vi "Set_positions_speeds.vi"(0 "m1":dbl, 1 "m2":dbl, 2 "m3":dbl, 3 "m4":dbl, 4 "m5":dbl, 5 "m6":dbl, 7 "error in (no error)":errorcluster, 9 "Speed m1":dbl, 11 "Speed m2":dbl, 13 "Speed m3":dbl, 15 "Speed m4":dbl, 17 "Speed m5":dbl, 19 "Speed m6":dbl) -> (27 "error out":errorcluster)   [LabVIEW 2017]
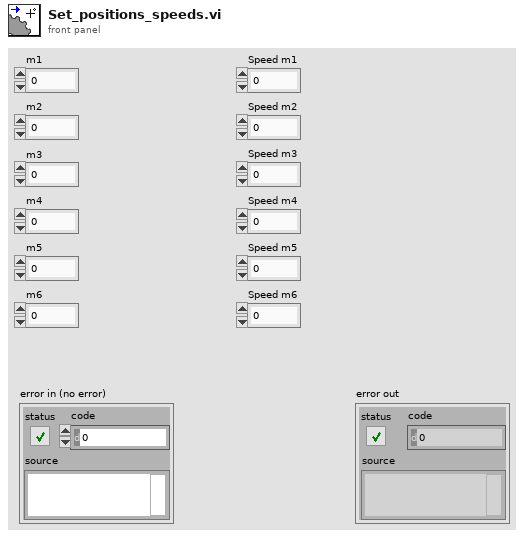
[diagram p1: front panel]
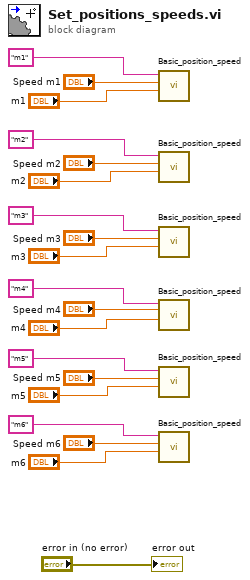
[diagram p0: block diagram]
diagram:
  n1 = call "Basic_position_speed.vi"("Position m?"="m1", "Speed m?"="Speed m1", "m?"="m1" ("string")) -> ()  [unwired: 8 in, 1 out]
  n2 = call "Basic_position_speed.vi"("Position m?"="m2", "Speed m?"="Speed m2", "m?"="m2" ("string")) -> ()  [unwired: 8 in, 1 out]
  n3 = call "Basic_position_speed.vi"("Position m?"="m3", "Speed m?"="Speed m3", "m?"="m3") -> ()  [unwired: 8 in, 1 out]
  n4 = call "Basic_position_speed.vi"("Position m?"="m4", "Speed m?"="Speed m4", "m?"="m4") -> ()  [unwired: 8 in, 1 out]
  n5 = call "Basic_position_speed.vi"("Position m?"="m5", "Speed m?"="Speed m5", "m?"="m5") -> ()  [unwired: 8 in, 1 out]
  n6 = call "Basic_position_speed.vi"("Position m?"="m6", "Speed m?"="Speed m6", "m?"="m6") -> ()  [unwired: 8 in, 1 out]
  "error out" <- "error in (no error)"
